vi "RT subVI - 1.vi"() -> ()   [LabVIEW 2016]
panel:
  out "fast counter":u16
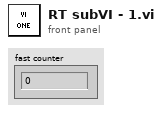
[diagram p1: front panel]
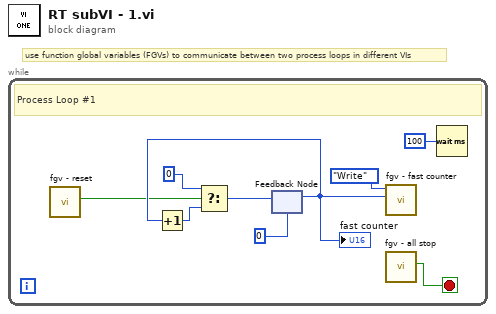
[diagram p0: block diagram]
diagram:
  # "use function global variables (FGVs) to communicate between two process loops in different VIs"
  n1 = while {
    stop <- w1 stop-if-true
    # "Process Loop #1"
    n2 = call "fgv - reset.vi"() -> ("Read Data"=w2:bool)  [unwired: 10 in, 1 out]
    n3 = feedback #1(u16 0) -> (w3:u16)
    "fast counter" <- w3
    n4 = Increment(x=w3) -> (x+1=w6:u16)
    n5 = Select(t=u16 0 ("f"), s=w2, f=w6) -> (s? t:f=w8:u16)
    n6 = feedback-in #1(w8) -> ()
    n7 = call "fgv - fast counter.vi"("Write Data (0)"=w3, "Operation"=enum16{"Read", "Write"}."Write") -> ()  [unwired: 8 in, 2 out]
    n8 = call "fgv - all stop.vi"() -> ("Read Data"=w1:bool)  [unwired: 10 in, 1 out]
    n9 = Wait (ms)(milliseconds to wait=u32 100) -> ()  [unwired: 1 out]
  }
